vi "AMI_Extrae_ZNB_Measure.vi"(10 "String":string="Spectrum from 1.0E+5 Hz to 1.0E+6 Hz, Bandwidth 25.00 Hz, 201 points, Power -20.00 dB") -> (1 "Array":string[](array[string]))   [LabVIEW 2017]
panel:
  # "Spectrum from 1.0E+5 Hz to 1.0E+6 Hz, Bandwidth 25.00 Hz, 201 points, Power -20.00 dB"
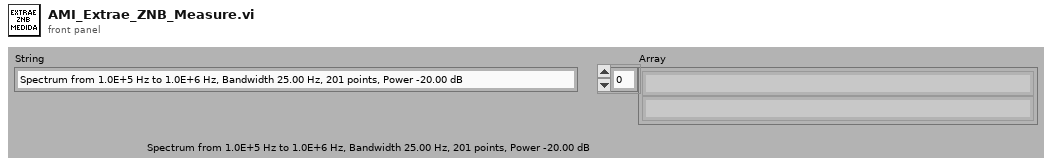
[diagram p1: front panel]
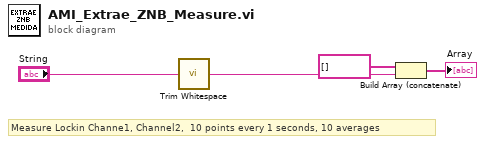
[diagram p0: block diagram]
diagram:
  # "Measure Lockin Channe1, Channel2,  10 points every 1 seconds, 10 averages"
  n1 = call <vilib>:"Trim Whitespace.vi"("string"="String") -> ("trimmed string"=w1:string)  [unwired: 1 in]
  n2 = Build Array (concatenate)(string[] [] ("Array I"), w1) -> (→"Array":string[])
